vi "탭웹브라우저(0).vi"() -> ()   [LabVIEW 2014]
panel:
  out "2":i32
  out "1":i32
  in  "정지":bool
  in  "탭 컨트롤":enum32{"페이지 1", "페이지 2"}(tab)
  in  "WebBrowser":refnum<k7>(container) caption="웹 브라우저"
  in  "WebBrowser 2":refnum<k7>(container) caption="웹 브라우저"
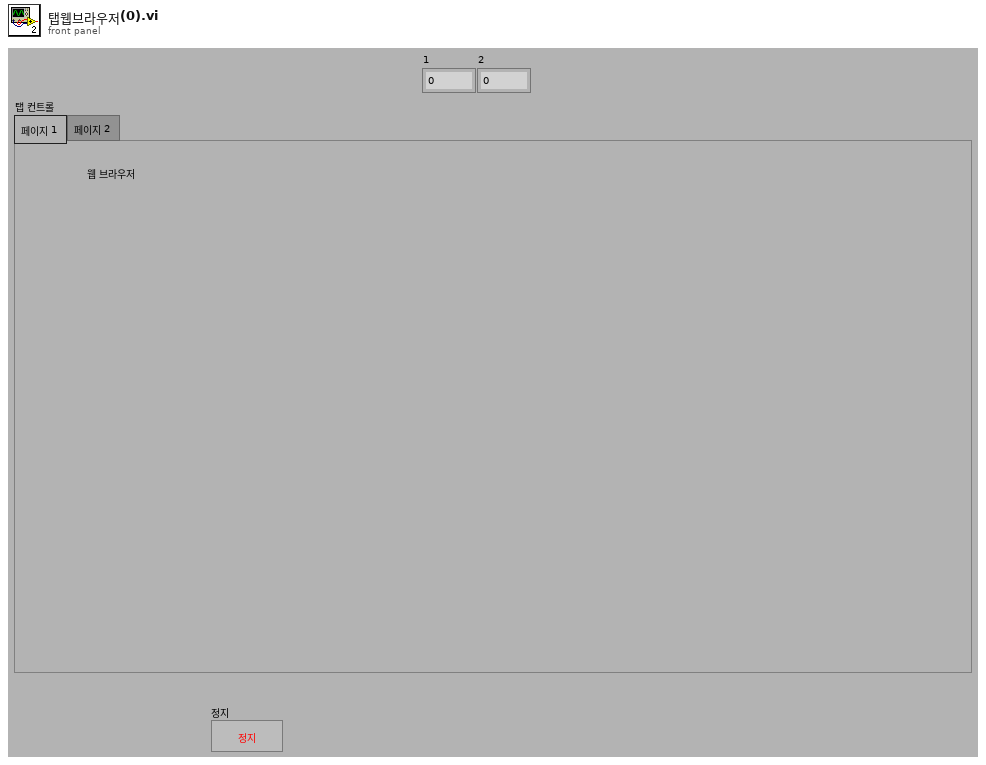
[diagram p1: front panel]
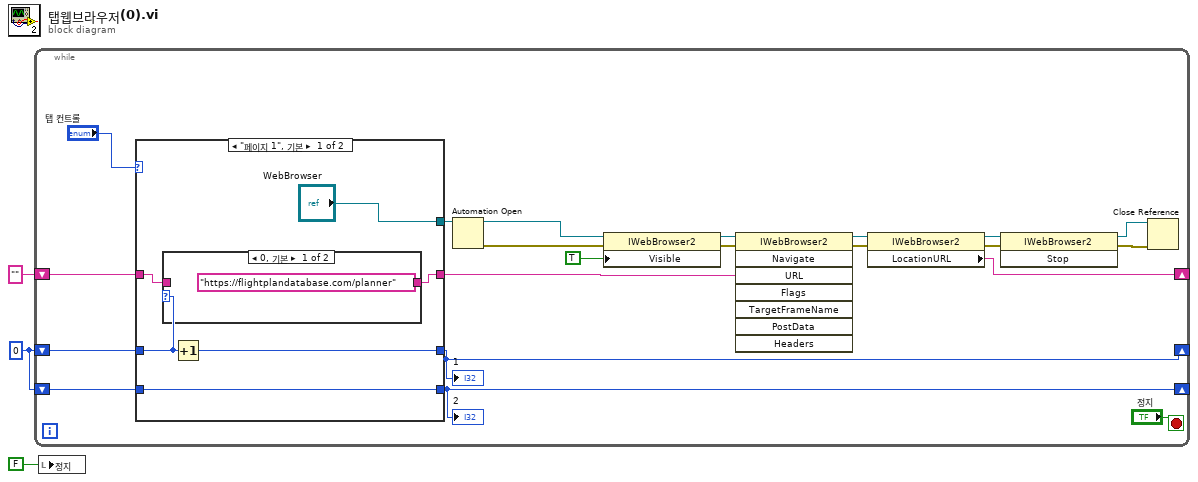
[diagram p0: block diagram]
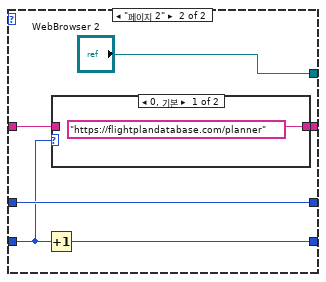
[diagram p3: hidden frame]
diagram:
  w2 = 0
  n1 = while {
    shift-right: [w15] -> _
    shift-left: "" ("LocationURL") -> [w14]
    shift-right: [w10] -> _
    shift-left: w2 -> [w11]
    shift-right: [w12] -> _
    shift-left: w2 -> [w13]
    stop <- "정지" stop-if-true
    n2 = case shown="\"페이지 1\", 기본" "탭 컨트롤" {
      tunnel: ["WebBrowser" "WebBrowser 2"] -> w19
      tunnel: [w29 w37] -> w21
      tunnel: w14 -> [w28 w35]
      tunnel: w13 -> [w25 w36]
      tunnel: [w27 w36] -> w12
      tunnel: w11 -> [w26 w33]
      tunnel: [w26 w34] -> w10
      frame "페이지 1", Default {
        n3 = case shown="0, 기본" w25 {
          tunnel: ["https://flightplandatabase.com/planner" w32] -> w29
          tunnel: w28 -> [_ w32]
          frame 0, Default {
          }
          frame 1.. {
          }
        }
        n4 = Increment(x=w25) -> (x+1=w27:i32)
      }
      frame "페이지 2" {
        n5 = Increment(x=w33) -> (x+1=w34:i32)
        n6 = case shown="0, 기본" w33 {
          tunnel: ["https://flightplandatabase.com/planner" w40] -> w37
          tunnel: w35 -> [_ w40]
          frame 0, Default {
          }
          frame 1.. {
          }
        }
      }
    }
    "1" <- w12
    "2" <- w10
    n7 = Automation Open(Automation Refnum=w19) -> (Automation Refnum=w18:refnum<k7>, error out=w17:errorcluster)  [unwired: 1 in, 2 out]
    n8 = property class="IWebBrowser2"(reference=w18, error in=w17, "Visible"=TRUE) -> (reference out=w22:refnum<k7>, error out=w23:errorcluster)
    n9 = invoke class="IWebBrowser2" method="Navigate"(reference=w22, error in=w23, "URL"=w21) -> (reference out=w9:refnum<k7>, error out=w8:errorcluster)  [unwired: 5 in, 6 out]
    n10 = property class="IWebBrowser2"(reference=w9, error in=w8) -> (reference out=w7:refnum<k7>, error out=w6:errorcluster, "LocationURL"=w15:string)
    n11 = invoke class="IWebBrowser2" method="Stop"(reference=w7, error in=w6) -> (reference out=w4:refnum<k7>, error out=w5:errorcluster)  [unwired: 1 in, 1 out]
    n12 = Close Reference(reference=w4, error in (no error)=w5) -> ()  [unwired: 1 out]
  }
  n13 = local write "정지"(FALSE ("정지")) -> ()
